vi "Main.vi"() -> ()   [LabVIEW 2018]
doc: "This template is for the Queued Message Handler design pattern.\n\nThe Event Handling Loop generates messages based on user interface actions.\n\nThe Message Handling Loop processes messages generated by the Event Handling Loop, or by other messages. The messages are string values, so new messages can be added easily to the Message Cases case structure in the Message Handling Loop. Each message cluster can also provide an optional value for Message Data, which is a variant that can be converted to whatever message-specific data is required."
uses:
  <vilib>/MakerHub/LINX/Private/Type Defs/LINX Ref.ctl
  <vilib>/MakerHub/LINX/Private/Type Defs/Platform.ctl
  <vilib>/MakerHub/LINX/Private/Type Defs/Interface.ctl
  <vilib>/MakerHub/LINX/Private/Device/Type Defs/LINX Device Config.ctl
  <vilib>/MakerHub/LINX/Private/Device/Type Defs/TCP Config.ctl
  <vilib>/MakerHub/LINX/Private/Device/Type Defs/Channels.ctl
  <vilib>/MakerHub/LINX/Public/Peripherals/Digital/Digital Write N Chans.vi
  <vilib>/MakerHub/LINX/Private/Local IO/LinxDigitalWrite.vi
  <vilib>/MakerHub/LINX/Public/Utilities/Check Channel.vi
  <vilib>/MakerHub/LINX/Public/Utilities/Open Serial.vi
  <vilib>/MakerHub/LINX/Private/Utilties/Generate Error.vi
  lib/Olympus IX BX Series/Olympus IX BX Series.lvlib
  <vilib>/MakerHub/LINX/LMH-LINX.lvlib
  lib/SOLA/LabVIEW 2015 Library (32bit)/LumencorDLL32/LumencorDLL32.lvlib
  lib/ANDOR/Andor SDK/AndorSDK.lvlib
  <vilib>/vision/NI_Vision_Development_Module.lvlib
  lib/tiff/LVTiffWriter/LVTiffWriter.lvlib
  <vilib>/MakerHub/LINX/Private/Device/Device.lvlib
  C:/Users/johan/Downloads/LabVIEW software/LabVIEW software/IX-81 Software/lib/tiff/LVTiffWriter/BitMiracle.LibTiff.NET.dll
  lib/tiff/LVTiffWriter/BitMiracle.LibTiff.NET.dll
panel:
  out "CalibFile":path
  in  "Messages":string
  in  "Desired Refresh Ratio":dbl format="%#_g %"
  out "Number of pump steps\n for the desired refresh ratio":dbl
  out "error IO":errorcluster
  out "TiffHandle":refnum<k24>
  in  "Image Name":string="TestIMG"
  out "Acq. Error Array":cluster{i32, string}[](array[cluster])
  in  "Single Image":bool
  out "Image":T1(plugin-control)
  in  "Exposure":sgl=50.0 format="%#_g ms"
  in  "Colormap":u16(ring) items=["Grey", "Hot"]
  in  "Format":u16(ring)=6
  in  "Path":path
  in  "Save Image":bool
  in  "Exposure 2":sgl=50.0 format="%#_g ms"
  in  "Filter":u16(ring) items=["UV ", "CFP", "GFP", "YFP", "RFP", "BF (empty)"]
  out "exposure out":sgl
  out "accumulate out":sgl
  out "kinetic out":sgl
  out "Camera Temperature":sgl format="%.2f °C"
  in  "Calibrate at Startup":bool
  out "Y Limits":dbl[](array[numeric]) caption="Y Limits [µm]" format="%#_12f"
  out "X Limits":dbl[](array[numeric]) caption="X Limits [µm]" format="%#_10f"
  out "Lower Limit":dbl
  out "Upper Limit":dbl
  in  "Focus [um]":dbl format="%.3f"
  in  "Intensity [%]":dbl(slide) scale=0.0..100.0 scale format="%.1f"
  in  "Light Source":u16(ring) items=["BF - Lamp", "SOLA"]
  in  "Prism Position (1: Bi)":enum16{"Bi", "Side"}(ring)=enum."Side"
  in  "Objective":enum16{"x 4", "x 10", "x 20", "x 40", "x 100"}(ring)=enum."x 10"
  in  "Lamp Type (0: Transmitted)":enum16{"Transmitted", "Reflected"}(ring)
  in  "Enable Lamp":bool
  in  "Shutter":bool
  in  "Microscope Settings":i32(listbox)
  out "Slide":u8(slide) scale=0.0..100.0
  in  "Valve Actuation":i32(listbox)
  in  "Configuration File Path":path
  in  "stop":bool
  out "error out":errorcluster
  in  "Position List":i32[](listbox)
  out "SOLA ID":u32
  out "TANGO ID":i32
  out "LINX Resource":T2={"IO"=enum."Remote", "Interface"=enum."TCP", "LINX Device Config"={"Interface"=enum."Serial", "COM Port"="COM13", "TCP Configuration"={"IP Address"="", "Port"=0}, "Device Family"=1, "Device ID"=1, "Device Name"="myRIO-1900", "TCP Ref"=refnum, "Channels"={"DI"=[0, 1, 2, 3, 4, 5, 6, 7, 8, 9, 10, 11, 12, 13, 14, 15, 16, 17, 18, 19, 20, 21, 22, 23, 24, 25, 26, 27, 28, 29, 30, 31, 32, 33, 34, 35, 36, 37, 38, 39, 40, 41, 42, 43, 44, 45, 46], "DO"=[0, 1, 2, 3, 4, 5, 6, 7, 8, 9, 10, 11, 12, 13, 14, 15, 16, 17, 18, 19, 20, 21, 22, 23, 24, 25, 26, 27, 28, 29, 30, 31, 32, 33, 34, 35, 36, 37, 38, 39, 40, 41, 42, 43, 44, 45, 46], "AI"=[0, 1, 2, 3, 4, 5, 6, 7, 8, 9, 10, 11], "AO"=[], "PWM"=[3, 5, 6, 9, 10], "QE"=[], "UART"=[0, 1], "I2C 2"=[0], "SPI"=[0], "CAN"=[], "Servo"=[], "AI Ref (V)"=0.0, "AI Resolution (Bits)"=0, "AO Ref (V)"=0.0, "AO Resolution (Bits)"=0}}}
  out "Tango Success":bool
  in  "TANGO COM Port":refnum<visa-resource-name>="COM4"
  in  "SOLA COM Port":refnum<visa-resource-name>="COM5"
  in  "Valve Port (Arduino)":refnum<visa-resource-name>="COM7"
  in  "IX 81 Port":refnum<visa-resource-name>="IX2-UCB"
  # "Initialization"
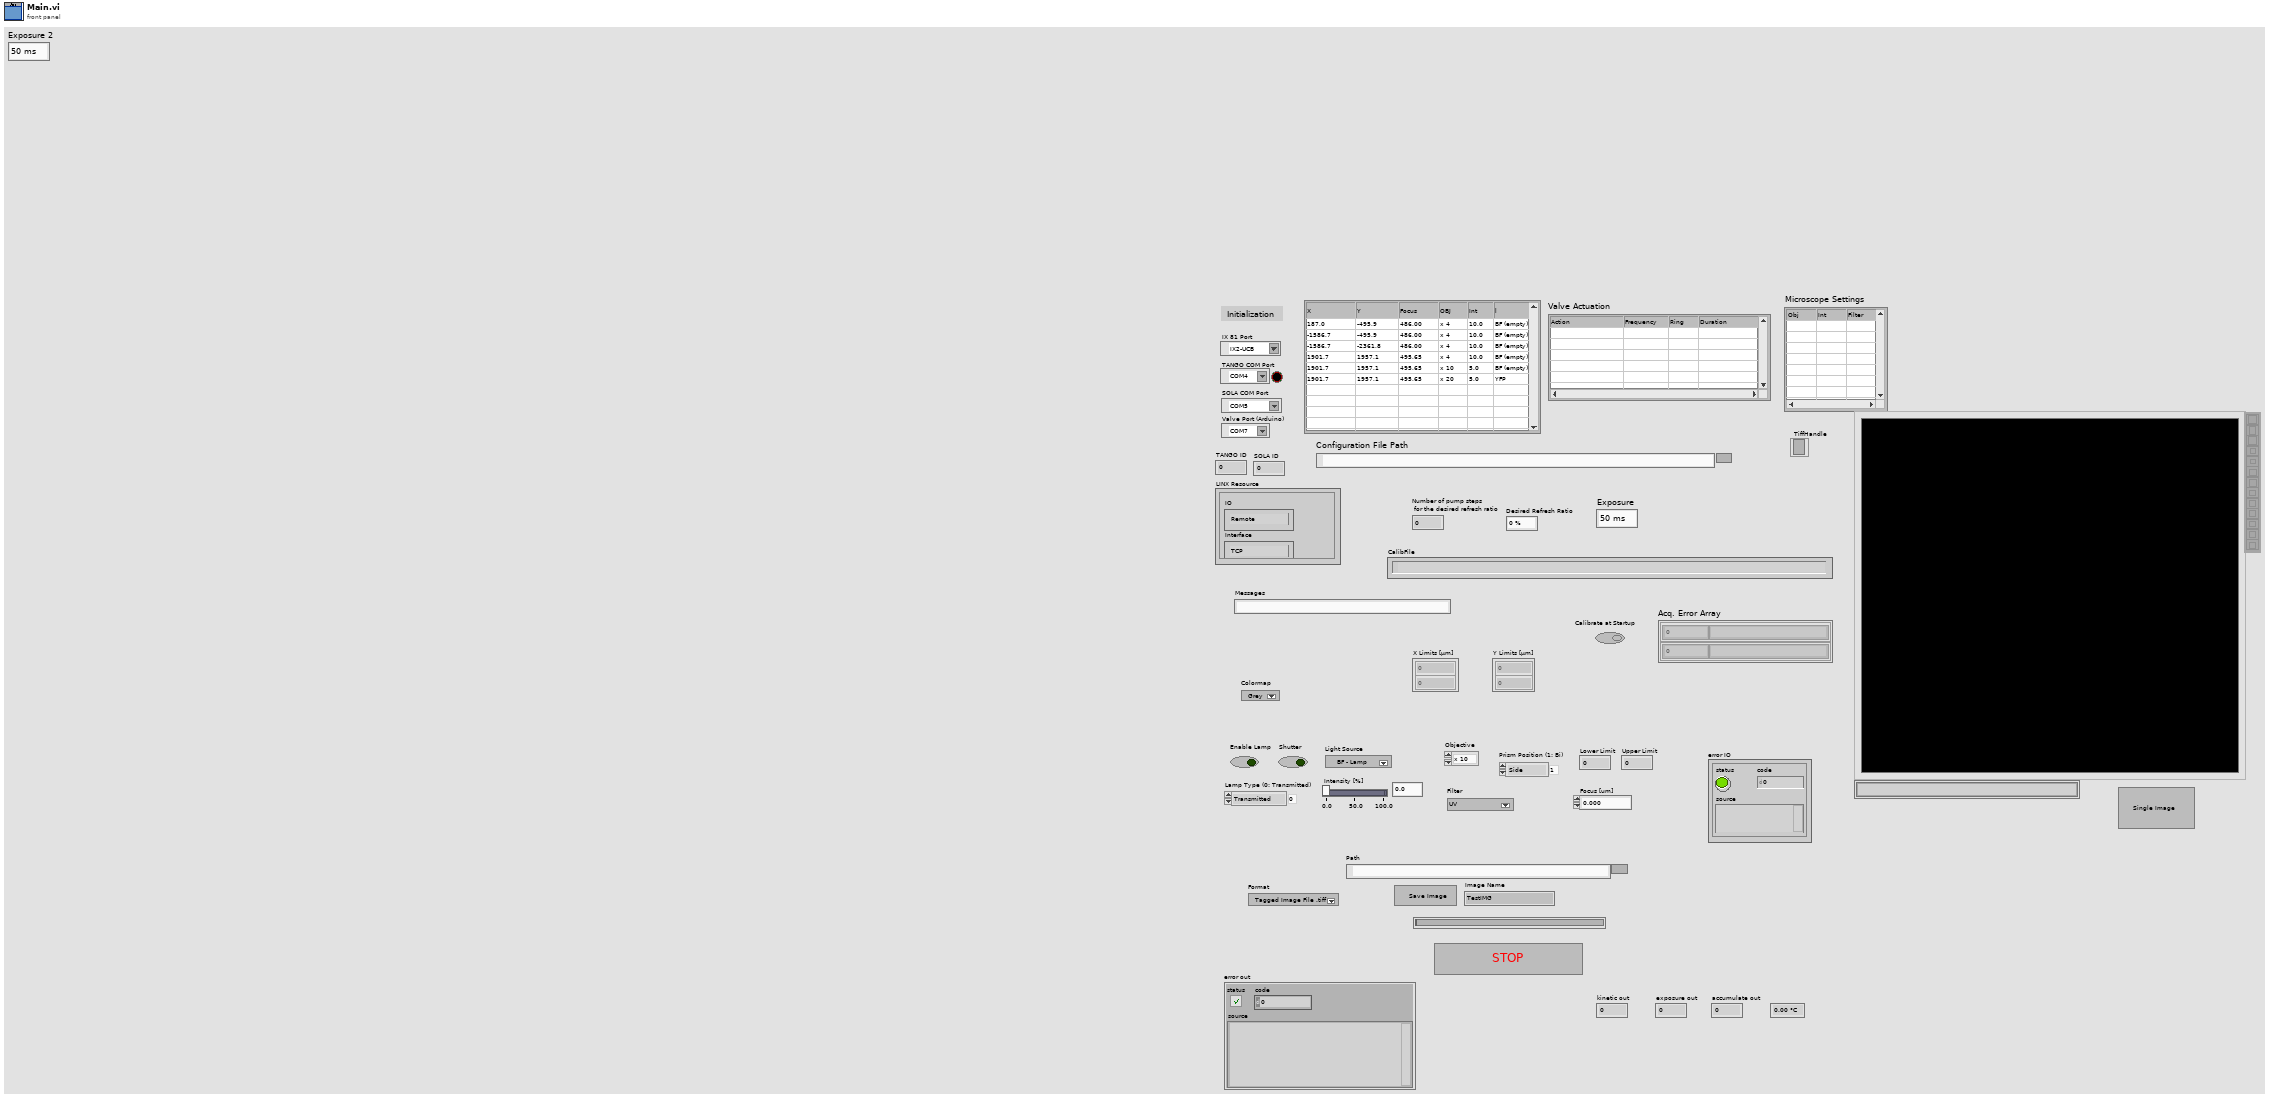
[diagram p1: front panel]
types:
  T1 = typedef "IMAQ Image.ctl" = refnum<image>
  T2 = typedef "LMH-LINX.lvlib/LINX Ref.ctl" = cluster{"IO":T3, "Interface":T4, "LINX Device Config":T5}
  T3 = typedef "LMH-LINX.lvlib/Platform.ctl" = enum16{"Remote", "Local"}
  T4 = typedef "LMH-LINX.lvlib/Interface.ctl" = enum16{"Serial", "TCP"}
  T5 = typedef "LMH-LINX.lvlib/Device.lvlib/LINX Device Config.ctl" = cluster{"Interface":T4, "COM Port":refnum<visa-resource-name>, "TCP Configuration":T6, "Device Family":u8, "Device ID":u8, "Device Name":string, "TCP Ref":refnum<k5>, "Channels":T7}
  T6 = typedef "LMH-LINX.lvlib/Device.lvlib/TCP Config.ctl" = cluster{"IP Address":string, "Port":u16}
  T7 = typedef "LMH-LINX.lvlib/Channels.ctl" = cluster{"DI":u8[], "DO":u8[], "AI":u8[], "AO":u8[], "PWM":u8[], "QE":u8[], "UART":u8[], "I2C 2":u8[], "SPI":u8[], "CAN":u8[], "Servo":u8[], "AI Ref (V)":dbl, "AI Resolution (Bits)":u8, "AO Ref (V)":dbl, "AO Resolution (Bits)":u8}
  T8 = enum16{"open", "replace", "create", "open or create", "replace or create", "replace or create with confirmation"}
  T9 = typedef "Image Type" = u32
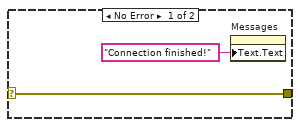
[diagram p2: hidden frame]
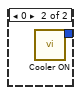
[diagram p3: hidden frame]
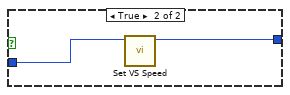
[diagram p4: hidden frame]
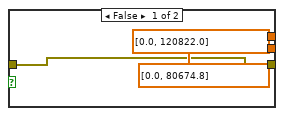
[diagram p5: hidden frame]
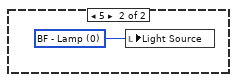
[diagram p6: hidden frame]
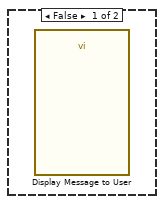
[diagram p8: hidden frame]
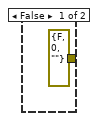
[diagram p12: hidden frame]
diagram:
  n1 = flat-sequence {
    tunnel: [w8] -> w5
    tunnel: w5 -> [w39]
    tunnel: [w38] -> w4
    tunnel: w4 -> [_]
    tunnel: [w442] -> w3
    tunnel: w3 -> [w474]
    tunnel: [w472] -> w2
    tunnel: [w471] -> w1
    tunnel: w2 -> [w477]
    tunnel: w1 -> [_]
    frame #0 {
      w28 = 2  # Device Number (1: Condensor, Objective Lamp,Shutter 2: Z-Motion, Autofocus)
      w31 = 1  # Device Number (1: Condensor, Objective Lamp,Shutter 2: Z-Motion, Autofocus)
      n2 = property on="SOLA COM Port" class="VISAName"() -> ("Text.Text"=w11:string)  [unwired: 2 in, 2 out]
      n3 = local read "IX 81 Port"() -> (w27:refnum<visa-resource-name>)
      n4 = local read "Valve Port (Arduino)"() -> (w26:refnum<visa-resource-name>)
      n5 = Scan From String(format string="COM%d", input string=w11) -> (output 1=w22:i32)  [unwired: 3 in, 3 out]
      n6 = Decrement(x=w22) -> (x-1=w21:i32)
      n7 = local read "TANGO COM Port"() -> (w15:refnum<visa-resource-name>)
      n8 = call "Initialize.vi"("dir"="C:\\Users\\e14user\\Documents\\LabVIEW software\\GitRepo\\lib\\ANDOR\\Libraries") -> ("function return"=w17:u32)  [unwired: 9 in, 1 out]
      n9 = call "Initialize.vi"("VISA Resource Name"=w27) -> ("VISA Resource Name Out"=w32:refnum<visa-resource-name>, "error out"=w33:errorcluster)  [unwired: 13 in]
      n10 = call "lm Init.vi"("LETypeStr"="SOLA", "ComPort"=w21) -> ("error out"=w19:errorcluster, "function return"=→"SOLA ID":u32)  [unwired: 7 in, 1 out]
      n11 = call "Login Device.vi"("error in (no error)"=w33, "Device Number (1)"=w31, "VISA Resource Name"=w32) -> ("error out"=w29:errorcluster, "VISA Resource Name Out"=w30:refnum<visa-resource-name>)  [unwired: 7 in]
      n12 = call "AndorCreaterErrorCluster.vi"() -> ("Array"=w12:cluster{i32, string}[])  [unwired: 11 in]
      n13 = call-poly <vilib>:"Open.vi"("Serial Port"=w26) -> ("Error Out"=w24:errorcluster, "LINX Resource"=→"LINX Resource":T2)  [unwired: 8 in, 1 out]
      n14 = call "Login Device.vi"("error in (no error)"=w29, "Device Number (1)"=w28, "VISA Resource Name"=w30) -> ("error out"=w25:errorcluster)  [unwired: 7 in, 1 out]
      n15 = call "AndorReturn2Error.vi"("Error List"=w12, "Camera return"=w17) -> ("error out"=w16:errorcluster)  [unwired: 8 in, 1 out]
      n16 = call "TangoConnect.vi"("Tango Com"=w15) -> ("error out"=w14:errorcluster, "success"=w13:bool, "plLSID out"=w7:i32)  [unwired: 7 in, 1 out]
      n17 = Merge Errors(w25, w24, w19, w14, w16) -> (w9:errorcluster)
      n18 = local write "TANGO ID"(w7) -> ()
      n19 = local write "Tango Success"(w13) -> ()
      n20 = case shown="Error" w9 {
        selector: w9 -> [w34 w37]
        tunnel: [w34 w37] -> w8
        frame No Error {
          n21 = property on="Messages" class="Str"("Text.Text"="Connection finished!") -> ()  [unwired: 2 in, 2 out]
        }
        frame Error {
          n22 = property on="Messages" class="Str"("Text.Text"="Connection did not work!\nTry restarting every single device.") -> ()  [unwired: 2 in, 2 out]
        }
      }
    }
    frame #1 {
      w104 = 0  # openingtime
      w102 = 0  # Auto Mode
      w101 = 1  # TTL High to open
      w103 = 0  # closingtime
      w100 = 0  # Internal Trigger
      w98 = 1  # Single Scan
      w99 = 4  # Image Read
      n23 = local read "IX 81 Port"() -> (w186:refnum<visa-resource-name>)
      n24 = local read "Calibrate at Startup"() -> (w122:bool)
      n25 = local write "Lower Limit"(10.0 ("Upper Limit")) -> ()
      n26 = call "Set Temperature.vi"("temperature"=-60) -> ()  [unwired: 10 in, 1 out]
      n27 = local write "Upper Limit"(3000000.0 ("default (0 I32)")) -> ()
      n28 = call "lm Color Level.vi"("error in (no error)"=w39, "str_Level"="0", "str_Color"="WHITE") -> ("error out"=w190:errorcluster, "str_Color out"=w191:string)  [unwired: 6 in, 1 out]
      n29 = case shown="True" w122 {
        tunnel: [w199 w206] -> w111
        tunnel: w39 -> [w199 w202]
        tunnel: [dbl[] [0.0, 80674.8] ("Y Limits") w205] -> w120
        tunnel: [dbl[] [0.0, 120822.0] ("X Limits") w204] -> w121
        frame False {
        }
        frame True {
          n30 = local read "TANGO ID"() -> (w203:i32)
          n31 = call "TangoCalibrate.vi"("error in (no error)"=w202, "plLSID in"=w203) -> ("error out"=w206:errorcluster, "X Limits"=w204:dbl[], "Y Limits"=w205:dbl[])  [unwired: 7 in]
        }
      }
      n32 = call "Set Active Objective.vi"("error in (no error)"=w39, "Objective Number (1)"=1, "Device Number (1)"=1, "VISA Resource Name"=w186) -> ("error out"=w137:errorcluster, "VISA Resource Name Out"=w138:refnum<visa-resource-name>)  [unwired: 6 in]
      n33 = call "lm Color Enable.vi"("error in (no error)"=w190, "str_State"="OFF", "str_Color"=w191) -> ("error out"=w112:errorcluster)  [unwired: 6 in, 2 out]
      n34 = call "OlympusQuery.vi"("error in (no error)"=w137, "String"="SW OFF", "VISA Resource Name In"=w138) -> ("error out"=w141:errorcluster, "VISA Resource Name Out"=w142:refnum<visa-resource-name>)  [unwired: 6 in, 1 out]
      n35 = call "Is Cooler On.vi"() -> ("function return"=w87:u32, "iCoolerStatus out"=w88:i32)  [unwired: 10 in]
      n36 = call "OlympusQuery.vi"("error in (no error)"=w141, "String"="LMPSW OFF", "VISA Resource Name In"=w142) -> ("error out"=w136:errorcluster, "VISA Resource Name Out"=w183:refnum<visa-resource-name>)  [unwired: 6 in, 1 out]
      n37 = case shown="1, Default" w88 {
        tunnel: [u32 20002 ("function return") w195] -> w86
        frame 1, Default {
        }
        frame 0 {
          n38 = call "Cooler ON.vi"() -> ("function return"=w195:u32)  [unwired: 11 in]
        }
      }
      n39 = call "Get VS Speed.vi"() -> ("speed out"=w107:sgl, "function return"=w74:u32)  [unwired: 10 in]
      n40 = call "Get Fastest Recommended VS Speed.vi"() -> ("function return"=w73:u32, "speed out"=w106:sgl, "index out"=w109:i32)  [unwired: 9 in]
      n41 = Greater Or Equal?(x=w106, y=w107) -> (x >= y?=w108:bool)
      n42 = call "OlympusQuery.vi"("error in (no error)"=w136, "String"="LMP?", "VISA Resource Name In"=w183) -> ("error out"=w134:errorcluster, "Result"=w144:string, "VISA Resource Name Out"=w182:refnum<visa-resource-name>)  [unwired: 6 in]
      n43 = call "AndorCreaterErrorCluster.vi"() -> ("Array"=w72:cluster{i32, string}[])  [unwired: 11 in]
      n44 = case shown="False" w108 {
        tunnel: w109 -> [_ w198]
        tunnel: [u32 20002 ("function return") w197] -> w75
        frame False {
        }
        frame True {
          n45 = call "Set VS Speed.vi"("index"=w198) -> ("function return"=w197:u32)  [unwired: 10 in]
        }
      }
      n46 = local write "Y Limits"(w120) -> ()
      n47 = local write "X Limits"(w121) -> ()
      n48 = call "AndorReturn2Error.vi"("Error List"=w72, "Camera return"=w87) -> ("error out"=w70:errorcluster, "Error List out"=w71:cluster{i32, string}[])  [unwired: 8 in]
      n49 = Decimal String To Number(string=w144, default (0L)=0.0 ("default (0 I32)")) -> (number=w146:dbl)  [unwired: 1 in, 1 out]
      n50 = local read "LINX Resource"() -> (w119:T2)
      n51 = call "AndorReturn2Error.vi"("error in (no error)"=w70, "Error List"=w71, "Camera return"=w86) -> ("error out"=w69:errorcluster, "Error List out"=w43:cluster{i32, string}[])  [unwired: 7 in]
      n52 = call "OlympusQuery.vi"("error in (no error)"=w134, "String"="SHUT1?", "VISA Resource Name In"=w182) -> ("error out"=w132:errorcluster, "Result"=w165:string, "VISA Resource Name Out"=w180:refnum<visa-resource-name>)  [unwired: 6 in]
      n53 = call "ArdnoValve2Linx.vi"("error in (no error)"=w39, "Valve (A1-C8),\n comma separated"="A1,A2,A3,A4,A5,A6,A7,A8,B1,B2,B3,B4,B5,B6,B7,B8,C1,C2,C3,C4,C5,C6,C7,C8" ("Valve (A1-C8),\n comma separated")) -> ("error out"=w117:errorcluster, "Array"=w116:bool[], "Array 2"=w115:i32[])  [unwired: 7 in]
      n54 = Divide(x=w146, y=1.2 ("x")) -> (x/y=w135:dbl)
      n55 = call-poly <vilib>:"Digital Write.vi"("Error In"=w117, "Values"=w116, "DO Channels"=w115, "LINX Resource"=w119) -> ("Error Out"=w113:errorcluster)  [unwired: 6 in, 1 out]
      n56 = local write "Intensity [%]"(w135) -> ()
      n57 = call "AndorReturn2Error.vi"("error in (no error)"=w69, "Error List"=w43, "Camera return"=w73) -> ("error out"=w68:errorcluster, "Error List out"=w44:cluster{i32, string}[])  [unwired: 7 in]
      n58 = Equal?(x=w165, y="OUT") -> (x = y?=w133:bool)
      n59 = call "AndorReturn2Error.vi"("error in (no error)"=w68, "Error List"=w44, "Camera return"=w74) -> ("error out"=w67:errorcluster, "Error List out"=w45:cluster{i32, string}[])  [unwired: 7 in]
      n60 = call "OlympusQuery.vi"("error in (no error)"=w132, "String"="LMPSEL?", "VISA Resource Name In"=w180) -> ("error out"=w129:errorcluster, "Result"=w163:string, "VISA Resource Name Out"=w130:refnum<visa-resource-name>)  [unwired: 6 in]
      n61 = call "Get Temperature F.vi"() -> ("function return"=w76:u32, "temperature out"=w105:sgl)  [unwired: 10 in]
      n62 = call "AndorReturn2Error.vi"("error in (no error)"=w67, "Error List"=w45, "Camera return"=w75) -> ("error out"=w66:errorcluster, "Error List out"=w46:cluster{i32, string}[])  [unwired: 7 in]
      n63 = local write "Shutter"(w133) -> ()
      n64 = Equal?(x=w163, y="DIA") -> (x = y?=w161:bool)
      n65 = local write "Camera Temperature"(w105) -> ()
      n66 = call "AndorReturn2Error.vi"("error in (no error)"=w66, "Error List"=w46, "Camera return"=w76) -> ("error out"=w65:errorcluster, "Error List out"=w47:cluster{i32, string}[])  [unwired: 7 in]
      n67 = call "Set Read Mode.vi"("mode"=w99) -> ("function return"=w77:u32)  [unwired: 10 in]
      n68 = call "OlympusQuery.vi"("error in (no error)"=w129, "String"="MU?", "VISA Resource Name In"=w130) -> ("error out"=w128:errorcluster, "Result"=w159:string, "VISA Resource Name Out"=w140:refnum<visa-resource-name>)  [unwired: 6 in]
      n69 = call "Set Shutter.vi"("openingtime"=w104, "closingtime"=w103, "mode"=w102, "typ"=w101) -> ("function return"=w78:u32)  [unwired: 7 in]
      n70 = Decimal String To Number(string=w159) -> (number=w158:i32)  [unwired: 2 in, 1 out]
      n71 = call "AndorReturn2Error.vi"("error in (no error)"=w65, "Error List"=w47, "Camera return"=w77) -> ("error out"=w64:errorcluster, "Error List out"=w48:cluster{i32, string}[])  [unwired: 7 in]
      n72 = Not(x=w161) -> (.not. x?=w160:bool)
      n73 = Boolean To (0,1)(Boolean=w160) -> (0, 1=w131:i16)
      n74 = call "AndorReturn2Error.vi"("error in (no error)"=w64, "Error List"=w48, "Camera return"=w78) -> ("error out"=w63:errorcluster, "Error List out"=w49:cluster{i32, string}[])  [unwired: 7 in]
      n75 = call "Set Trigger Mode.vi"("mode"=w100) -> ("function return"=w79:u32)  [unwired: 10 in]
      n76 = Decrement(x=w158) -> (x-1=w139:i32)
      n77 = call "OlympusQuery.vi"("error in (no error)"=w128, "String"="OB 2", "VISA Resource Name In"=w140) -> ("error out"=w127:errorcluster, "VISA Resource Name Out"=w175:refnum<visa-resource-name>)  [unwired: 6 in, 1 out]
      n78 = local write "Lamp Type (0: Transmitted)"(w131) -> ()
      n79 = local write "Filter"(w139) -> ()
      n80 = call "Set Acquisition Mode.vi"("mode"=w98) -> ("function return"=w80:u32)  [unwired: 10 in]
      n81 = call "AndorReturn2Error.vi"("error in (no error)"=w63, "Error List"=w49, "Camera return"=w79) -> ("error out"=w62:errorcluster, "Error List out"=w50:cluster{i32, string}[])  [unwired: 7 in]
      n82 = case shown="0, Default" w139 {
        frame 0, Default {
          w207 = u16 1 items=["BF - Lamp", "SOLA"] ("Light Source")
          n83 = local write "Light Source"(w207) -> ()
        }
        frame 5 {
          w208 = u16 0 items=["BF - Lamp", "SOLA"] ("Light Source")
          n84 = local write "Light Source"(w208) -> ()
        }
      }
      n85 = call "AndorReturn2Error.vi"("error in (no error)"=w62, "Error List"=w50, "Camera return"=w80) -> ("error out"=w61:errorcluster, "Error List out"=w51:cluster{i32, string}[])  [unwired: 7 in]
      n86 = call "OlympusQuery.vi"("error in (no error)"=w127, "String"="PRISM?", "VISA Resource Name In"=w175) -> ("error out"=w126:errorcluster, "Result"=w157:string, "VISA Resource Name Out"=w174:refnum<visa-resource-name>)  [unwired: 6 in]
      n87 = Decimal String To Number(string=w157) -> (number=w156:i32)  [unwired: 2 in, 1 out]
      n88 = call "Set Frame Transfer Mode.vi"("mode"=1) -> ("function return"=w81:u32)  [unwired: 10 in]
      n89 = Decrement(x=w156) -> (x-1=w125:i32)
      n90 = call "OlympusQuery.vi"("error in (no error)"=w126, "Device Number\n(1: -Condensor\n     - Objective\n     - Lamp\n     - Shutter\n2: - Z-Motion\n   - Autofocus)"=2 ("Device Number\n(1: -Condensor\n     - Objective\n     - Lamp\n     - Shutter\n2: - Z-Motion\n   - Autofocus)"), "String"="FARLMT 10", "VISA Resource Name In"=w174) -> ("error out"=w171:errorcluster, "VISA Resource Name Out"=w172:refnum<visa-resource-name>)  [unwired: 5 in, 1 out]
      n91 = call "AndorReturn2Error.vi"("error in (no error)"=w61, "Error List"=w51, "Camera return"=w81) -> ("error out"=w60:errorcluster, "Error List out"=w52:cluster{i32, string}[])  [unwired: 7 in]
      n92 = local read "Exposure"() -> (w94:sgl)
      n93 = local write "Prism Position (1: Bi)"(w125) -> ()
      n94 = call "Set Number Accumulations.vi"("number"=1) -> ("function return"=w82:u32)  [unwired: 10 in]
      n95 = call "OlympusQuery.vi"("error in (no error)"=w171, "Device Number\n(1: -Condensor\n     - Objective\n     - Lamp\n     - Shutter\n2: - Z-Motion\n   - Autofocus)"=2 ("Device Number\n(1: -Condensor\n     - Objective\n     - Lamp\n     - Shutter\n2: - Z-Motion\n   - Autofocus)"), "String"="NEARLMT 3000000", "VISA Resource Name In"=w172) -> ("error out"=w168:errorcluster, "VISA Resource Name Out"=w169:refnum<visa-resource-name>)  [unwired: 5 in, 1 out]
      n96 = call "AndorReturn2Error.vi"("error in (no error)"=w60, "Error List"=w52, "Camera return"=w82) -> ("error out"=w59:errorcluster, "Error List out"=w53:cluster{i32, string}[])  [unwired: 7 in]
      n97 = call "Set Number Kinetics.vi"("number"=1) -> ("function return"=w83:u32)  [unwired: 10 in]
      n98 = Divide(x=w94, y=sgl 1000.0) -> (x/y=w93:sgl)
      n99 = call "AndorReturn2Error.vi"("error in (no error)"=w59, "Error List"=w53, "Camera return"=w83) -> ("error out"=w58:errorcluster, "Error List out"=w54:cluster{i32, string}[])  [unwired: 7 in]
      n100 = call "Set Exposure Time.vi"("time"=w93) -> ("function return"=w84:u32)  [unwired: 10 in]
      n101 = call "OlympusQuery.vi"("error in (no error)"=w168, "Device Number\n(1: -Condensor\n     - Objective\n     - Lamp\n     - Shutter\n2: - Z-Motion\n   - Autofocus)"=2 ("Device Number\n(1: -Condensor\n     - Objective\n     - Lamp\n     - Shutter\n2: - Z-Motion\n   - Autofocus)"), "String"="POS?", "VISA Resource Name In"=w169) -> ("error out"=w150:errorcluster, "Result"=w151:string, "VISA Resource Name Out"=w149:refnum<visa-resource-name>)  [unwired: 5 in]
      n102 = call "AndorReturn2Error.vi"("error in (no error)"=w58, "Error List"=w54, "Camera return"=w84) -> ("error out"=w57:errorcluster, "Error List out"=w55:cluster{i32, string}[])  [unwired: 7 in]
      n103 = call "Get Acquisition Timings.vi"() -> ("kinetic out"=w91:sgl, "accumulate out"=w89:sgl, "exposure out"=w90:sgl, "function return"=w85:u32)  [unwired: 8 in]
      n104 = Decimal String To Number(string=w151, default (0L)=0.0 ("default (0 I32)")) -> (number=w41:dbl)  [unwired: 1 in, 1 out]
      n105 = local write "exposure out"(w90) -> ()
      n106 = local write "accumulate out"(w89) -> ()
      n107 = local write "kinetic out"(w91) -> ()
      n108 = call "AndorReturn2Error.vi"("error in (no error)"=w57, "Error List"=w55, "Camera return"=w85) -> ("error out"=w56:errorcluster)  [unwired: 7 in, 1 out]
      n109 = call "Configure Jog.vi"("VISA Resource Name"=w149, "Device Number (1)"=2, "Enabled (False)"=TRUE, "error in (no error)"=w150) -> ("error out"=w114:errorcluster)  [unwired: 10 in, 1 out]
      n110 = Divide(x=w41, y=1000.0) -> (x/y=w40:dbl)
      n111 = Merge Errors(w114, w113, w112, w111, w56) -> (w38:errorcluster)
      n112 = local write "Focus [um]"(w40) -> ()
    }
    frame #2 {
      n113 = Two Button Dialog(message="Do you want to calibrate the pumps now?") -> (T button?=w209:bool)  [unwired: 2 in]
      n114 = case shown="True" w209 {
        frame False {
        }
        frame True {
          n115 = flat-sequence {
            frame #0 {
              n116 = Open/Create/Replace File(operation (0:open)=T8."create", access (0:read/write)=enum16{"read/write", "read-only", "write-only"}."read/write") -> (refnum out=w213:refnum<file>, error out=w214:errorcluster)  [unwired: 4 in, 1 out]
              n117 = Close File(refnum=w213, error in=w214) -> (path=w212:path)  [unwired: 1 out]
              "CalibFile" <- w212
              n118 = call "tiffOpenForWrite.vi"("Path"=w212) -> ("TiffOut"=→"TiffHandle":refnum<k24>)  [unwired: 10 in]
            }
            frame #1 {
              w222 = u16 1 items=["BF - Lamp", "SOLA"] ("Light Source")
              n119 = local write "Light Source"(w222) -> ()
              n120 = property on="Filter" class="Ring (strict)"() -> ("Strings []"=w221:string[])  [unwired: 2 in, 2 out]
              n121 = call "Exposure Time check"() -> ("Color"=w220:string, "Exposure Time"=w223:dbl)  [unwired: 16 in, 2 out]
              n122 = Array Size(array=w221) -> (size(s)=w218:i32)
              n123 = for {
                N: w218 -> [_]
                tunnel: w221 -> [w234] mode=indexing
                tunnel: w220 -> [w233]
                tunnel: [w232] -> w217
                i -> [w232]
                stop <- w235 stop-if-true
                n124 = Equal?(x=w233, y=w234) -> (x = y?=w235:bool)
              }
              n125 = flat-sequence {
                tunnel: [w236] -> w224
                tunnel: w223 -> [w237]
                tunnel: w224 -> [w246]
                frame #0 {
                  n126 = while {
                    tunnel: w237 -> [w238]
                    tunnel: [w238] -> w236
                    stop <- w239 stop-if-true
                    n127 = call "Get Status.vi"() -> ("function return"=w245:u32, "status out"=w242:i32)  [unwired: 10 in]
                    n128 = Equal?(x=20073 ("status out"), y=w242) -> (x = y?=w241:bool)
                    n129 = Equal?(x=w245, y=20002 ("x")) -> (x = y?=w240:bool)
                    n130 = And(x=w241, y=w240) -> (x .and. y?=w239:bool)
                  }
                }
                frame #1 {
                  n131 = Divide(x=w246, y=sgl 1000.0) -> (x/y=w248:dbl)
                  n132 = call "Set Exposure Time.vi"("time"=w248) -> ()  [unwired: 10 in, 1 out]
                }
              }
              n133 = Less?(x=w217, y=w218) -> (x < y?=w219:bool)
              n134 = case shown="True" w219 {
                tunnel: w217 -> [_ w228]
                frame False {
                  n135 = call "Display Message to User"() -> ()  [unwired: 10 in, 2 out]
                }
                frame True {
                  n136 = Increment(x=w228) -> (x+1=w227:i32)
                  n137 = Number To Decimal String(number=w227) -> (decimal integer string=w229:string)  [unwired: 1 in]
                  n138 = call <vilib>:"Space Constant.vi"() -> ("String"=w231:string)
                  n139 = local read "IX 81 Port"() -> (w225:refnum<visa-resource-name>)
                  n140 = Concatenate Strings("MU", w231, w229) -> (w226:string)
                  n141 = call "OlympusQuery.vi"("String"=w226, "VISA Resource Name In"=w225) -> ()  [unwired: 7 in, 3 out]
                }
              }
            }
            frame #2 {
              n142 = flat-sequence {
                tunnel: TRUE ("NewVal") -> [w257]
                tunnel: [w257] -> w252
                tunnel: [w261] -> w251
                tunnel: w252 -> [w261]
                tunnel: w249 -> [w262]
                tunnel: w251 -> [w263]
                frame #0 {
                  w255 = 1  # Single Scan
                  w256 = 4  # Image Read
                  n143 = call "Set Number Accumulations.vi"("number"=1) -> ()  [unwired: 10 in, 1 out]
                  n144 = call "Set Read Mode.vi"("mode"=w256) -> ()  [unwired: 10 in, 1 out]
                  n145 = call "Set Acquisition Mode.vi"("mode"=w255) -> ()  [unwired: 10 in, 1 out]
                  n146 = call "Set Number Kinetics.vi"("number"=1) -> ()  [unwired: 10 in, 1 out]
                }
                frame #1 {
                  n147 = local read "Exposure"() -> (w258:sgl)
                  n148 = Divide(x=w258, y=sgl 1000.0) -> (x/y=w260:sgl)
                  n149 = call "Set Exposure Time.vi"("time"=w260) -> ()  [unwired: 10 in, 1 out]
                }
                frame #2 {
                  n150 = case shown="True" w263 {
                    tunnel: w262 -> [_ w273]
                    frame False {
                    }
                    frame True {
                      n151 = flat-sequence {
                        tunnel: w273 -> [w274]
                        tunnel: [w276] -> w272
                        tunnel: [w275] -> w271
                        tunnel: w272 -> [w278]
                        tunnel: w271 -> [w279]
                        tunnel: [w279] -> w270
                        tunnel: [w278] -> w269
                        tunnel: w270 -> [w294]
                        tunnel: w269 -> [w293]
                        tunnel: [w294] -> w268
                        tunnel: [w293] -> w267
                        tunnel: [w289] -> w266
                        tunnel: [w290] -> w265
                        tunnel: w268 -> [w298]
                        tunnel: w267 -> [w296]
                        tunnel: w266 -> [w297]
                        tunnel: w265 -> [w300]
                        tunnel: [w300] -> w264
                        tunnel: w264 -> [w316]
                        frame #0 {
                          n152 = call "Start Acquisition.vi"() -> ("function return"=w277:u32)  [unwired: 11 in]
                          n153 = call "ConvertErrCodeToMessage.vi"("function return"=w277, "Array"=w274) -> ("Element Return"=w275:cluster{i32, string}, "Array out"=w276:cluster{i32, string}[])  [unwired: 8 in]
                        }
                        frame #1 {
                          n154 = while {
                            stop <- w280 stop-if-true
                            n155 = call "Get Status.vi"() -> ("function return"=w286:u32, "status out"=w283:i32)  [unwired: 10 in]
                            n156 = Equal?(x=20073 ("status out"), y=w283) -> (x = y?=w282:bool)
                            n157 = Equal?(x=w286, y=20002 ("x")) -> (x = y?=w281:bool)
                            n158 = And(x=w282, y=w281) -> (x .and. y?=w280:bool)
                          }
                        }
                        frame #2 {
                          n159 = Square(x=1024) -> (x^2=w287:i32)
                          n160 = Initialize Array(i16 0 ("element"), w287) -> (w288:i16[])
                          n161 = call "Get Most Recent Image16.vi"("size"=w287, "arr"=w288) -> ("function return"=w289:u32, "arr out"=w290:u16[])  [unwired: 7 in, 1 out]
                        }
                        frame #3 {
                          n162 = call "ConvertErrCodeToMessage.vi"("function return"=w297, "Array"=w296) -> ("Element Return"=w299:cluster{i32, string})  [unwired: 8 in, 1 out]
                          n163 = Build Array(w299, w298) -> (w295:cluster{i32, string}[])
                          n164 = local write "Acq. Error Array"(w295) -> ()
                        }
                        frame #4 {
                          w319 = u32 2 items=["Zero Order", "Bi-Linear", "Quadratic", "Cubic Spline"] ("Interpolation Type")
                          w318 = T9 1 items=["Grayscale (U8)", "Grayscale (I16)", "Grayscale (SGL)", "Complex (CSG)", "RGB (U32)", "HSL (U32)", "RGB (U64)", "Grayscale (U16)"] ("Image Type")
                          w317 = 1024 ("dimension size")
                          n165 = local read "Image Name"() -> (w315:string)
                          n166 = Reshape Array(w316, w317, w317) -> (w321:u16[][])
                          n167 = call "IMAQ Create"("Image Name"=w315, "Image Type"=w318) -> ("New Image"=w320:T1)  [unwired: 3 in, 1 out]
                          n168 = property on="Image" class="ImageControl"() -> ("Image Area Height"=w312:u32, "Image Area Width"=w313:u32)  [unwired: 2 in, 2 out]
                          n169 = call "IMAQ ArrayToImage"("Image Pixels (I16)"=w321, "Image"=w320) -> ("Image Out"=w314:T1)  [unwired: 8 in, 1 out]
                          n170 = call "IMAQ GetImageSize"("Image"=w314) -> ("Y Resolution"=w306:i32, "X Resolution"=w309:i32)  [unwired: 3 in, 1 out]
                          n171 = Divide(x=w306, y=w312) -> (x/y=w322:dbl)
                          n172 = Divide(x=w309, y=w313) -> (x/y=w323:dbl)
                          n173 = Max & Min(x=w322, y=w323) -> (max(x,y)=w311:dbl, min(x,y)=w307:dbl)
                          n174 = Divide(x=w309, y=w311) -> (x/y=w310:dbl)
                          n175 = Divide(x=w306, y=w307) -> (x/y=w308:dbl)
                          n176 = local read "TiffHandle"() -> (w301:refnum<k24>)
                          n177 = call "IMAQ Resample"("X Resolution"=w310, "Y Resolution"=w308, "Interpolation Type"=w319, "Image Src"=w314) -> ("Image Dst Out"=w305:T1)  [unwired: 6 in, 1 out]
                          n178 = call "tiffWriteImaqToTiff.vi"("Multipage"=cluster{"Page":i32, "TotalPages":i32} {"Page"=11, "TotalPages"=1}, "ImaqIn"=w305, "TiffIn"=w301) -> ("ImaqOut"=w303:T1, "TiffOut"=w302:refnum<k24>)  [unwired: 7 in]
                          n179 = local write "Image"(w303) -> ()
                          n180 = local write "TiffHandle"(w302) -> ()
                        }
                      }
                    }
                  }
                }
              }
              n181 = call "AndorCreaterErrorCluster.vi"() -> ("Array"=w249:cluster{i32, string}[])  [unwired: 11 in]
            }
            frame #3 {
              n182 = Two Button Dialog(message="Start dilution. Please load the fluorophore now") -> (T button?=w325:bool)  [unwired: 2 in]
              n183 = case shown="True" w325 {
                frame False {
                }
                frame True {
                  n184 = flat-sequence {
                    tunnel: [w329] -> w328
                    tunnel: w328 -> [w334]
                    tunnel: [w334] -> w327
                    tunnel: w327 -> [w338]
                    tunnel: [w336] -> w326
                    frame #0 {
                      n185 = local read "LINX Resource"() -> (w333:T2)
                      n186 = call "ArdnoFlush.vi"("Open?"=FALSE, "Single / Multivalve?"=FALSE, "Channel"=u32 1, "LINX Resource"=w333) -> ("LINX Resource out"=w329:T2)  [unwired: 6 in, 1 out]
                    }
                    frame #1 {
                      n187 = Wait (ms)(milliseconds to wait=u32 60000) -> ()  [unwired: 1 out]
                    }
                    frame #2 {
                      (unwired) u32 1 ("Channel")
                      n188 = call "ArdnoFlush.vi"("Open?"=TRUE, "Single / Multivalve?"=FALSE, "LINX Resource"=w338) -> ("LINX Resource out"=w336:T2)  [unwired: 7 in, 1 out]
                    }
                  }
                  n189 = while {
                    tunnel: w326 -> [w343]
                    i -> [w340]
                    stop <- w344 continue-if-true
                    n190 = flat-sequence {
                      tunnel: w343 -> [w352]
                      tunnel: [w348] -> w342
                      tunnel: [w347] -> w341
                      tunnel: w342 -> [w357]
                      tunnel: w341 -> [w356]
                      tunnel: w340 -> [w358]
                      frame #0 {
                        n191 = call "ArdnoFeed.vi"("LINX Resource"=w352, "Single / Multivalve?"=FALSE, "Channel"=u32 1, "Feed Cycles"=15, "Frequency"=u32 10) -> ("LINX Resource out"=w348:T2, "error out"=w347:errorcluster)  [unwired: 9 in]
                      }
                      frame #1 {
                        n192 = call "ArdnoPump.vi"("LINX Resource"=w357, "Pump Cycles"=4, "Pump Frequency"=50, "error in (no error)"=w356, "Single/\nMultiring?"=FALSE ("Single/\nMultiring?")) -> ()  [unwired: 2 out]
                      }
                      frame #2 {
                        n193 = flat-sequence {
                          tunnel: TRUE ("NewVal") -> [w367]
                          tunnel: [w367] -> w362
                          tunnel: [w371] -> w361
                          tunnel: w362 -> [w371]
                          tunnel: w359 -> [w373]
                          tunnel: w361 -> [w374]
                          tunnel: w358 -> [w372]
                          frame #0 {
                            w365 = 1  # Single Scan
                            w366 = 4  # Image Read
                            n194 = call "Set Number Accumulations.vi"("number"=1) -> ()  [unwired: 10 in, 1 out]
                            n195 = call "Set Acquisition Mode.vi"("mode"=w365) -> ()  [unwired: 10 in, 1 out]
                            n196 = call "Set Read Mode.vi"("mode"=w366) -> ()  [unwired: 10 in, 1 out]
                            n197 = call "Set Number Kinetics.vi"("number"=1) -> ()  [unwired: 10 in, 1 out]
                          }
                          frame #1 {
                            n198 = local read "Exposure"() -> (w368:sgl)
                            n199 = Divide(x=w368, y=sgl 1000.0) -> (x/y=w370:sgl)
                            n200 = call "Set Exposure Time.vi"("time"=w370) -> ()  [unwired: 10 in, 1 out]
                          }
                          frame #2 {
                            n201 = case shown="True" w374 {
                              tunnel: w373 -> [_ w385]
                              tunnel: w372 -> [_ w375]
                              frame False {
                              }
                              frame True {
                                n202 = flat-sequence {
                                tunnel: w385 -> [w386]
                                tunnel: [w388] -> w384
                                tunnel: [w387] -> w383
                                tunnel: w384 -> [w390]
                                tunnel: w383 -> [w391]
                                tunnel: [w391] -> w382
                                tunnel: [w390] -> w381
                                tunnel: w382 -> [w406]
                                tunnel: w381 -> [w405]
                                tunnel: [w406] -> w380
                                tunnel: [w405] -> w379
                                tunnel: [w401] -> w378
                                tunnel: [w402] -> w377
                                tunnel: w380 -> [w410]
                                tunnel: w379 -> [w408]
                                tunnel: w378 -> [w409]
                                tunnel: w377 -> [w412]
                                tunnel: [w412] -> w376
                                tunnel: w376 -> [w433]
                                tunnel: w375 -> [w413]
                                frame #0 {
                                n203 = call "Start Acquisition.vi"() -> ("function return"=w389:u32)  [unwired: 11 in]
                                n204 = call "ConvertErrCodeToMessage.vi"("function return"=w389, "Array"=w386) -> ("Element Return"=w387:cluster{i32, string}, "Array out"=w388:cluster{i32, string}[])  [unwired: 8 in]
                                }
                                frame #1 {
                                n205 = while {
                                stop <- w392 stop-if-true
                                n206 = call "Get Status.vi"() -> ("function return"=w398:u32, "status out"=w395:i32)  [unwired: 10 in]
                                n207 = Equal?(x=20073 ("status out"), y=w395) -> (x = y?=w394:bool)
                                n208 = Equal?(x=w398, y=20002 ("x")) -> (x = y?=w393:bool)
                                n209 = And(x=w394, y=w393) -> (x .and. y?=w392:bool)
                                }
                                }
                                frame #2 {
                                n210 = Square(x=1024) -> (x^2=w399:i32)
                                n211 = Initialize Array(i16 0 ("element"), w399) -> (w400:i16[])
                                n212 = call "Get Most Recent Image16.vi"("size"=w399, "arr"=w400) -> ("function return"=w401:u32, "arr out"=w402:u16[])  [unwired: 7 in, 1 out]
                                }
                                frame #3 {
                                n213 = call "ConvertErrCodeToMessage.vi"("function return"=w409, "Array"=w408) -> ("Element Return"=w411:cluster{i32, string})  [unwired: 8 in, 1 out]
                                n214 = Build Array(w411, w410) -> (w407:cluster{i32, string}[])
                                n215 = local write "Acq. Error Array"(w407) -> ()
                                }
                                frame #4 {
                                w436 = u32 2 items=["Zero Order", "Bi-Linear", "Quadratic", "Cubic Spline"] ("Interpolation Type")
                                w435 = T9 1 items=["Grayscale (U8)", "Grayscale (I16)", "Grayscale (SGL)", "Complex (CSG)", "RGB (U32)", "HSL (U32)", "RGB (U64)", "Grayscale (U16)"] ("Image Type")
                                w434 = 1024 ("dimension size")
                                n216 = Add(x=w413, y=2) -> (x+y=w415:i32)
                                n217 = local read "Image Name"() -> (w432:string)
                                n218 = Reshape Array(w433, w434, w434) -> (w438:u16[][])
                                n219 = call "IMAQ Create"("Image Name"=w432, "Image Type"=w435) -> ("New Image"=w437:T1)  [unwired: 3 in, 1 out]
                                n220 = property on="Image" class="ImageControl"() -> ("Image Area Height"=w429:u32, "Image Area Width"=w430:u32)  [unwired: 2 in, 2 out]
                                n221 = call "IMAQ ArrayToImage"("Image Pixels (I16)"=w438, "Image"=w437) -> ("Image Out"=w431:T1)  [unwired: 8 in, 1 out]
                                n222 = call "IMAQ GetImageSize"("Image"=w431) -> ("Y Resolution"=w423:i32, "X Resolution"=w426:i32)  [unwired: 3 in, 1 out]
                                n223 = Divide(x=w423, y=w429) -> (x/y=w439:dbl)
                                n224 = Divide(x=w426, y=w430) -> (x/y=w440:dbl)
                                n225 = Max & Min(x=w439, y=w440) -> (max(x,y)=w428:dbl, min(x,y)=w424:dbl)
                                n226 = Divide(x=w426, y=w428) -> (x/y=w427:dbl)
                                n227 = Divide(x=w423, y=w424) -> (x/y=w425:dbl)
                                n228 = Bundle By Name(cluster=cluster{"Page":i32, "TotalPages":i32} {"Page"=11, "TotalPages"=1} ("Multipage"), "TotalPages"=11, "Page"=w415) -> (w417:cluster{"Page":i32, "TotalPages":i32})
                                n229 = local read "TiffHandle"() -> (w419:refnum<k24>)
                                n230 = call "IMAQ Resample"("X Resolution"=w427, "Y Resolution"=w425, "Interpolation Type"=w436, "Image Src"=w431) -> ("Image Dst Out"=w422:T1)  [unwired: 6 in, 1 out]
                                n231 = call "tiffWriteImaqToTiff.vi"("Multipage"=w417, "ImaqIn"=w422, "TiffIn"=w419) -> ("ImaqOut"=w421:T1, "TiffOut"=w420:refnum<k24>)  [unwired: 7 in]
                                n232 = local write "Image"(w421) -> ()
                                n233 = local write "TiffHandle"(w420) -> ()
                                }
                                }
                              }
                            }
                          }
                        }
                        n234 = call "AndorCreaterErrorCluster.vi"() -> ("Array"=w359:cluster{i32, string}[])  [unwired: 11 in]
                      }
                    }
                    n235 = Less?(x=w340, y=10.0) -> (x < y?=w344:bool)
                  }
                }
              }
            }
          }
        }
      }
    }
    frame #3 {
      w445 = u32 20002  # DRV Return Success
      n236 = local read "TiffHandle"() -> (w441:refnum<k24>)
      n237 = call "Shut Down.vi"() -> ("function return"=w447:u32)  [unwired: 11 in]
      n238 = Not Equal?(x=w445, y=w447) -> (x != y?=w446:bool)
      n239 = call "AndorCreaterErrorCluster.vi"() -> ("Array"=w459:cluster{i32, string}[])  [unwired: 11 in]
      n240 = case shown="True" w446 {
        tunnel: w447 -> [_ w470]
        tunnel: w459 -> [_ w469]
        tunnel: [errorcluster {"status"=FALSE, "code"=0, "source"=""} ("error constant") w464] -> w458
        frame False {
        }
        frame True {
          n241 = call "ConvertErrCodeToMessage.vi"("function return"=w470, "Array"=w469) -> ("Element Return"=w468:cluster{i32, string})  [unwired: 8 in, 1 out]
          n242 = Unbundle(w468) -> (w466:i32, w467:string)
          n243 = Bundle By Name(cluster=errorcluster {"status"=FALSE, "code"=0, "source"=""} ("error constant"), "status"=TRUE, "code"=w466, "source"=w467) -> (w464:errorcluster)
        }
      }
      n244 = call "tiffClose.vi"("Tiff in"=w441) -> ()  [unwired: 10 in, 1 out]
      n245 = local read "IX 81 Port"() -> (w452:refnum<visa-resource-name>)
      n246 = call "Logout Device.vi"("Device Number (1)"=1, "VISA Resource Name"=w452) -> ("error out"=w451:errorcluster, "VISA Resource Name Out"=w449:refnum<visa-resource-name>)  [unwired: 8 in]
      n247 = local read "LINX Resource"() -> (w455:T2)
      n248 = local read "TANGO ID"() -> (w461:i32)
      n249 = local read "SOLA ID"() -> (w457:u32)
      n250 = call "Logout Device.vi"("error in (no error)"=w451, "Device Number (1)"=2, "VISA Resource Name"=w449) -> ("error out"=w450:errorcluster, "VISA Resource Name Out"=w448:refnum<visa-resource-name>)  [unwired: 7 in]
      n251 = call <vilib>:"Close.vi"("VISA Resource Name"=w448, "error in (no error)"=w450) -> ("error out"=w453:errorcluster)  [unwired: 13 in]
      n252 = call <vilib>:"Close.vi"("LINX Resource"=w455) -> ("Error Out"=w454:errorcluster)  [unwired: 10 in]
      n253 = call "lm Shut Down.vi"("hSerial"=w457) -> ("error out"=w456:errorcluster)  [unwired: 9 in, 1 out]
      n254 = call "Disconnect.vi"("lLSID"=w461) -> ("error out"=w460:errorcluster)  [unwired: 1 in]
      n255 = Merge Errors(w453, w454, w456, w460, w458) -> (w442:errorcluster)
    }
    frame #4 {
      n256 = script code="%% The aim of this script is to perform the calibration of the labview\n%  software with regards to the dilution volume as efficiently as possible\n%  requiring minimal input from the user. \n\n%% Set paths for Scripts and Functions\naddpath C:\\Users\\johan\\Downloads\\LabVIEW software\\LabVIEW software\\IX-81 Software\\Calibration\naddpath C:\\Users\\Nikon\\Desktop\\Matlab_Calibration_Script\\20170421_CalibrationScript_V2\n\n\n%% Select the correct .Tiff file:\n[fileName,pathName,filterIndex] = uigetfile(\"*.tif\");\nimg = loadTiffFast([pathName,fileName]);\n\n%% Provide the Initial Concentration of Fluorophore\ncellConcentration = inputdlg({'Input Initial Fluorophore Concentration:'});\ninitialConcentration = str2double(cellConcentration{1,1});\n\n%% Set the intensity range with which to view all images during ROI selection\ndesiredIntensity = selectIntensity(img(:, :, 2));\nintensityRange = [0, desiredIntensity];\n\n%% ROI selection for all chambers\n% A figure will be shown of the first image taken by the microscope at each\n% of the locations of interest within the microfluidic device. Using the\n% cursor, select an ROI (Region of Interest) where the fluorescence\n% intensity will be determined. This area should fall within the boundaries\n% of the microfluidic flow channel. Draw the area by selecting the corners\n% of a polygon (left mouse click) and accept the polygon by\n% double-clicking within the borders of the polygon. \n[xCoordinates, yCoordinates] = regionOfInterestDetermination(img, intensityRange);\n\n%% Determine the intensities of the ROI within all images\nintensities = intensityDetermination(img, xCoordinates, yCoordinates);\n\n%% Plot the intensity curves and view the refresh ratio\n[final_Refresh_Ratio, refreshPerReactor] = plotIntensityCurves(intensities);\n% RR1 = refreshPerReactor(1,1)\n% RR2 = refreshPerReactor(2,1)\n% RR3 = refreshPerReactor(3,1)\n% RR4 = refreshPerReactor(4,1)\n% RR5 = refreshPerReactor(5,1)\n% RR6 = refreshPerReactor(6,1)\n% RR7 = refreshPerReactor(7,1)\n% RR8 = refreshPerReactor(8,1)\n\n%% This is the end of the script."("??"=w474) -> ("??"=→"error IO":errorcluster, "refreshPerReactor"=w472:dbl, "finalRefreshRatio"=w471:dbl)
    }
    frame #5 {
      n257 = Divide(x="Desired Refresh Ratio", y=w477) -> (x/y=w479:dbl)
      n258 = Multiply(x=15.0, y=w479) -> (x*y=w478:dbl)
      n259 = Round To Nearest(number=w478) -> (nearest integer value=→"Number of pump steps\n for the desired refresh ratio":dbl)
    }
  }
